vi "write_PES_data.vi"(0 "Img-Bgd Data":i16[][](array[numeric]), 2 "Path":path, 7 "Img Data":i16[][](array[numeric]), 11 "Bgd Data":i16[][](array[numeric]), 12 "i01 Data":sgl[][](array[numeric]), 14 "i02 Data":sgl[][](array[numeric])) -> ()   [LabVIEW 2023]
uses:
  <vilib>/Utility/file.llb/Write To Spreadsheet File (I64).vi
  <vilib>/Utility/file.llb/Write To Spreadsheet File (DBL).vi
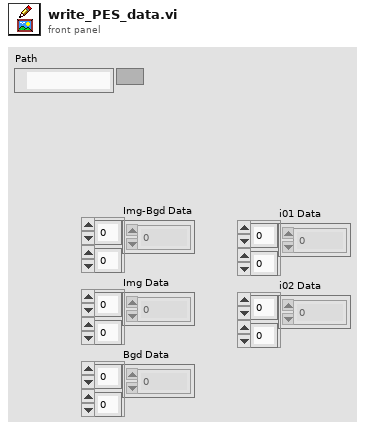
[diagram p1: front panel]
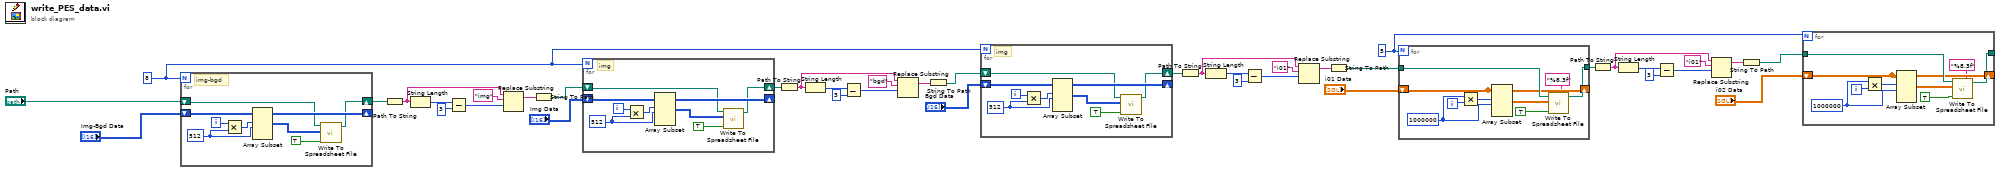
[diagram p0: block diagram]
diagram:
  w3 = 5
  w13 = 8
  n1 = for {
    N: w13 -> [_]
    shift-right: [w47] -> _
    shift-left: "Img-Bgd Data" -> [w47]
    shift-right: [w46] -> w36
    shift-left: "Path" -> [w45]
    i -> [w42]
    w44 = 512 ("length")
    # "img-bgd"
    n2 = Multiply(x=w42, y=w44) -> (x*y=w43:i32)
    n3 = Array Subset(array=w47, index (row)=w43, length (row)=w44) -> (w48:i16[][])  [unwired: 2 in]
    n4 = call-poly <vilib>:"Write To Spreadsheet File.vi"("append to file? (new file:F)"=TRUE, "2D data"=w48, "file path (dialog if empty)"=w45) -> ("new file path (Not A Path if cancelled)"=w46:path)  [unwired: 5 in]
  }
  n5 = Path To String(path=w36) -> (string=w35:string)
  n6 = String Length(string=w35) -> (length=w38:i32)
  n7 = Subtract(x=w38, y=3) -> (x-y=w40:i32)
  n8 = Replace Substring(3:w40, 4:"img" ("substring (\"\")"), 5:w35) -> (1:w34:string)  [unwired: 1 in, 1 out]
  n9 = String To Path(string=w34) -> (path=w32:path)
  n10 = for {
    N: w13 -> [_]
    shift-right: [w55] -> _
    shift-left: "Img Data" -> [w55]
    shift-right: [w54] -> w26
    shift-left: w32 -> [w53]
    i -> [w50]
    w52 = 512 ("length")
    # "img"
    n11 = Multiply(x=w50, y=w52) -> (x*y=w51:i32)
    n12 = Array Subset(array=w55, index (row)=w51, length (row)=w52) -> (w56:i16[][])  [unwired: 2 in]
    n13 = call-poly <vilib>:"Write To Spreadsheet File.vi"("append to file? (new file:F)"=TRUE, "2D data"=w56, "file path (dialog if empty)"=w53) -> ("new file path (Not A Path if cancelled)"=w54:path)  [unwired: 5 in]
  }
  n14 = Path To String(path=w26) -> (string=w28:string)
  n15 = String Length(string=w28) -> (length=w30:i32)
  n16 = Subtract(x=w30, y=3) -> (x-y=w25:i32)
  n17 = Replace Substring(3:w25, 4:"bgd" ("substring (\"\")"), 5:w28) -> (1:w27:string)  [unwired: 1 in, 1 out]
  n18 = String To Path(string=w27) -> (path=w23:path)
  n19 = for {
    N: w13 -> [_]
    shift-right: [w63] -> _
    shift-left: "Bgd Data" -> [w63]
    shift-right: [w62] -> w15
    shift-left: w23 -> [w61]
    i -> [w58]
    w60 = 512 ("length")
    # "img"
    n20 = Multiply(x=w58, y=w60) -> (x*y=w59:i32)
    n21 = Array Subset(array=w63, index (row)=w59, length (row)=w60) -> (w64:i16[][])  [unwired: 2 in]
    n22 = call-poly <vilib>:"Write To Spreadsheet File.vi"("append to file? (new file:F)"=TRUE, "2D data"=w64, "file path (dialog if empty)"=w61) -> ("new file path (Not A Path if cancelled)"=w62:path)  [unwired: 5 in]
  }
  n23 = Path To String(path=w15) -> (string=w19:string)
  n24 = String Length(string=w19) -> (length=w21:i32)
  n25 = Subtract(x=w21, y=3) -> (x-y=w17:i32)
  n26 = Replace Substring(3:w17, 4:"i01" ("substring (\"\")"), 5:w19) -> (1:w18:string)  [unwired: 1 in, 1 out]
  n27 = String To Path(string=w18) -> (path=w14:path)
  n28 = for {
    N: w3 -> [_]
    tunnel: w14 -> [w73]
    shift-right: [w68] -> _
    shift-left: "i01 Data" -> [w68]
    tunnel: [w66] -> w5
    i -> [w71]
    w69 = u32 1000000
    n29 = Multiply(x=w69, y=w71) -> (x*y=w70:u32)
    n30 = Array Subset(array=w68, index (row)=w70, length (row)=w69) -> (w72:sgl[][])  [unwired: 2 in]
    n31 = call-poly <vilib>:"Write To Spreadsheet File.vi"("format (%.3f)"="%8.3f", "append to file? (new file:F)"=TRUE, "2D data"=w72, "file path (dialog if empty)"=w73) -> ("new file path (Not A Path if cancelled)"=w66:path)  [unwired: 4 in]
  }
  n32 = Path To String(path=w5) -> (string=w9:string)
  n33 = String Length(string=w9) -> (length=w11:i32)
  n34 = Subtract(x=w11, y=3) -> (x-y=w7:i32)
  n35 = Replace Substring(3:w7, 4:"i01" ("substring (\"\")"), 5:w9) -> (1:w8:string)  [unwired: 1 in, 1 out]
  n36 = String To Path(string=w8) -> (path=w4:path)
  n37 = for {
    N: w3 -> [_]
    tunnel: w4 -> [w82]
    shift-right: [w77] -> _
    shift-left: "i02 Data" -> [w77]
    tunnel: [w75] -> _
    i -> [w80]
    w78 = u32 1000000
    n38 = Multiply(x=w78, y=w80) -> (x*y=w79:u32)
    n39 = Array Subset(array=w77, index (row)=w79, length (row)=w78) -> (w81:sgl[][])  [unwired: 2 in]
    n40 = call-poly <vilib>:"Write To Spreadsheet File.vi"("format (%.3f)"="%8.3f", "append to file? (new file:F)"=TRUE, "2D data"=w81, "file path (dialog if empty)"=w82) -> ("new file path (Not A Path if cancelled)"=w75:path)  [unwired: 4 in]
  }
